vi "ZoneBlue to ZoneRed.vi"   [LabVIEW 2019]
uses:
  Global Var.vi
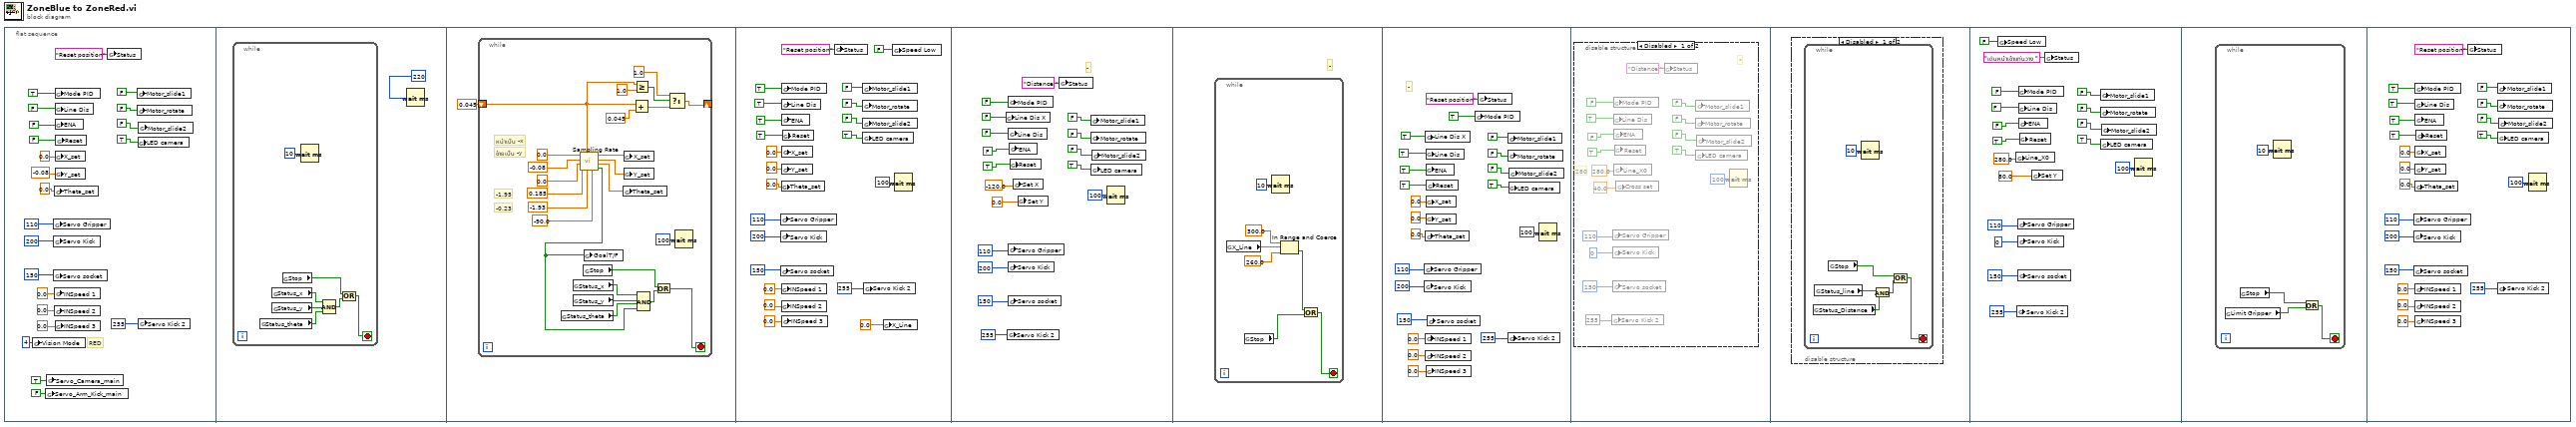
[diagram p0: block diagram]
diagram:
  n1 = flat-sequence {
    frame #0 {
      # "RED"
      n2 = global write "Global Var.vi" "Vision Mode"(i16 4 ("Vision Mode")) -> ()
      n3 = global write "Global Var.vi" "Servo_Arm_Kick_main"(FALSE ("Mode PID")) -> ()
      n4 = global write "Global Var.vi" "Servo_Camera_main"(TRUE ("Mode PID")) -> ()
      n5 = global write "Global Var.vi" "Servo Gripper"(u8 110 ("Servo Camera")) -> ()
      n6 = global write "Global Var.vi" "Servo Kick"(u8 200 ("Servo Camera")) -> ()
      n7 = global write "Global Var.vi" "Servo socket"(u8 150 ("Servo Camera")) -> ()
      n8 = global write "Global Var.vi" "Theta_set"(0.0 ("Theta_set")) -> ()
      n9 = global write "Global Var.vi" "INSpeed 1"(0.0 ("X_set")) -> ()
      n10 = global write "Global Var.vi" "INSpeed 2"(0.0 ("Y_set")) -> ()
      n11 = global write "Global Var.vi" "Mode PID"(TRUE ("Mode PID")) -> ()
      n12 = global write "Global Var.vi" "Line Dis"(FALSE ("Mode PID")) -> ()
      n13 = global write "Global Var.vi" "ENA"(FALSE ("ENA")) -> ()
      n14 = global write "Global Var.vi" "X_set"(0.0 ("X_set")) -> ()
      n15 = global write "Global Var.vi" "Y_set"(-0.08 ("Y_set")) -> ()
      n16 = global write "Global Var.vi" "INSpeed 3"(0.0 ("Theta_set")) -> ()
      n17 = global write "Global Var.vi" "Reset"(FALSE ("ENA")) -> ()
      n18 = global write "Global Var.vi" "Status"("Reset position" ("Status")) -> ()
      n19 = global write "Global Var.vi" "Motor_slide1"(FALSE ("Mode PID")) -> ()
      n20 = global write "Global Var.vi" "Motor_rotate"(FALSE ("ENA")) -> ()
      n21 = global write "Global Var.vi" "LED camera"(TRUE ("LED camera")) -> ()
      n22 = global write "Global Var.vi" "Motor_slide2"(FALSE ("ENA")) -> ()
      n23 = global write "Global Var.vi" "Servo Kick 2"(u8 255 ("Servo Camera")) -> ()
    }
    frame #1 {
      n24 = while {
        stop <- w26 stop-if-true
        n25 = global read "Global Var.vi" "Status_theta"() -> (w28:bool)
        n26 = global read "Global Var.vi" "Status_x"() -> (w29:bool)
        n27 = global read "Global Var.vi" "Status_y"() -> (w30:bool)
        n28 = global read "Global Var.vi" "Stop"() -> (w24:bool)
        n29 = Wait (ms)(milliseconds to wait=u32 10) -> ()  [unwired: 1 out]
        n30 = Compound Arithmetic op=AND(w29, w30, w28) -> (w25:bool)
        n31 = Or(x=w24, y=w25) -> (x .or. y?=w26:bool)
      }
      n32 = Wait (ms)(milliseconds to wait=u32 220) -> ()  [unwired: 1 out]
    }
    frame #2 {
      n33 = while {
        shift-right: [w34] -> _
        shift-left: 0.045 -> [w32]
        stop <- w51 stop-if-true
        # "-0.23"
        # "-1.95"
        # "ซ้ายเป็น -y"
        # "หน้าเป็น -x"
        n34 = global read "Global Var.vi" "Status_theta"() -> (w53:bool)
        n35 = global read "Global Var.vi" "Status_x"() -> (w54:bool)
        n36 = global read "Global Var.vi" "Status_y"() -> (w55:bool)
        n37 = call "Sampling Rate.vi"("input a1"=-90.0, "input y1"=-1.93, "T(0-1)"=w32, "input x1"=0.185, "input a0"=0.0, "input y0"=-0.08, "input x0"=0.0) -> ("GoalT/F"=w39:bool, "a_output"=w46:dbl, "y_output"=w47:dbl, "x_output"=w48:dbl)  [unwired: 1 in]
        n38 = global read "Global Var.vi" "Stop"() -> (w49:bool)
        n39 = global write "Global Var.vi" "GoalT/F"(w39) -> ()
        n40 = global write "Global Var.vi" "Theta_set"(w46) -> ()
        n41 = global write "Global Var.vi" "X_set"(w48) -> ()
        n42 = global write "Global Var.vi" "Y_set"(w47) -> ()
        n43 = Add(x=w32, y=0.045) -> (x+y=w37:dbl)
        n44 = Greater Or Equal?(x=w32, y=1.0) -> (x >= y?=w36:bool)
        n45 = Compound Arithmetic op=AND(w54, w55, w53, w39) -> (w50:bool)
        n46 = Or(x=w49, y=w50) -> (x .or. y?=w51:bool)
        n47 = Select(t=1.0, s=w36, f=w37) -> (s? t:f=w34:dbl)
        n48 = Wait (ms)(milliseconds to wait=u32 100) -> ()  [unwired: 1 out]
      }
    }
    frame #3 {
      n49 = global write "Global Var.vi" "Servo Gripper"(u8 110 ("Servo Camera")) -> ()
      n50 = global write "Global Var.vi" "Servo Kick"(u8 200 ("Servo Camera")) -> ()
      n51 = global write "Global Var.vi" "Servo socket"(u8 150 ("Servo Camera")) -> ()
      n52 = global write "Global Var.vi" "Theta_set"(0.0 ("Theta_set")) -> ()
      n53 = global write "Global Var.vi" "INSpeed 1"(0.0 ("X_set")) -> ()
      n54 = global write "Global Var.vi" "INSpeed 2"(0.0 ("Y_set")) -> ()
      n55 = global write "Global Var.vi" "Mode PID"(TRUE ("Mode PID")) -> ()
      n56 = global write "Global Var.vi" "Line Dis"(TRUE ("Mode PID")) -> ()
      n57 = global write "Global Var.vi" "ENA"(TRUE ("ENA")) -> ()
      n58 = global write "Global Var.vi" "X_set"(0.0 ("X_set")) -> ()
      n59 = global write "Global Var.vi" "Y_set"(0.0 ("Y_set")) -> ()
      n60 = global write "Global Var.vi" "INSpeed 3"(0.0 ("Theta_set")) -> ()
      n61 = global write "Global Var.vi" "Reset"(TRUE ("ENA")) -> ()
      n62 = global write "Global Var.vi" "Status"("Reset position" ("Status")) -> ()
      n63 = global write "Global Var.vi" "Motor_slide1"(FALSE ("Mode PID")) -> ()
      n64 = global write "Global Var.vi" "Motor_rotate"(FALSE ("ENA")) -> ()
      n65 = global write "Global Var.vi" "Motor_slide2"(FALSE ("ENA")) -> ()
      n66 = global write "Global Var.vi" "LED camera"(TRUE ("LED camera")) -> ()
      n67 = global write "Global Var.vi" "Servo Kick 2"(u8 255 ("Servo Camera")) -> ()
      n68 = global write "Global Var.vi" "X_Line"(0.0 ("X_set")) -> ()
      n69 = global write "Global Var.vi" "Speed Low"(FALSE ("LED camera")) -> ()
      n70 = Wait (ms)(milliseconds to wait=u32 100) -> ()  [unwired: 1 out]
    }
    frame #4 {
      # "-"
      n71 = global write "Global Var.vi" "Line Dis X"(FALSE ("Mode PID")) -> ()
      n72 = global write "Global Var.vi" "Servo Kick 2"(u8 255 ("Servo Camera")) -> ()
      n73 = global write "Global Var.vi" "Mode PID"(FALSE ("Mode PID")) -> ()
      n74 = global write "Global Var.vi" "Servo Gripper"(u8 110 ("Servo Camera")) -> ()
      n75 = global write "Global Var.vi" "Servo Kick"(u8 200 ("Servo Camera")) -> ()
      n76 = global write "Global Var.vi" "Servo socket"(u8 150 ("Servo Camera")) -> ()
      n77 = global write "Global Var.vi" "Line Dis"(FALSE ("Mode PID")) -> ()
      n78 = global write "Global Var.vi" "ENA"(FALSE ("ENA")) -> ()
      n79 = global write "Global Var.vi" "Reset"(TRUE ("ENA")) -> ()
      n80 = global write "Global Var.vi" "Set X"(-120.0 ("Y_set")) -> ()
      n81 = global write "Global Var.vi" "Set Y"(0.0 ("Y_set")) -> ()
      n82 = global write "Global Var.vi" "Status"("Distance " ("Status")) -> ()
      n83 = global write "Global Var.vi" "Motor_slide1"(FALSE ("Mode PID")) -> ()
      n84 = global write "Global Var.vi" "Motor_rotate"(FALSE ("ENA")) -> ()
      n85 = global write "Global Var.vi" "LED camera"(TRUE ("LED camera")) -> ()
      n86 = global write "Global Var.vi" "Motor_slide2"(FALSE ("ENA")) -> ()
      n87 = Wait (ms)(milliseconds to wait=u32 100) -> ()  [unwired: 1 out]
    }
    frame #5 {
      # "-"
      n88 = while {
        stop <- w100 stop-if-true
        n89 = global read "Global Var.vi" "X_Line"() -> (w98:dbl)
        n90 = global read "Global Var.vi" "Stop"() -> (w99:bool)
        n91 = Wait (ms)(milliseconds to wait=u32 10) -> ()  [unwired: 1 out]
        n92 = In Range and Coerce(upper limit=300.0, x=w98, lower limit=260.0) -> (In Range?=w95:bool)  [unwired: 1 out]
        n93 = Or(x=w95, y=w99) -> (x .or. y?=w100:bool)
      }
    }
    frame #6 {
      # "-"
      n94 = global write "Global Var.vi" "Servo Gripper"(u8 110 ("Servo Camera")) -> ()
      n95 = global write "Global Var.vi" "Servo Kick"(u8 200 ("Servo Camera")) -> ()
      n96 = global write "Global Var.vi" "Line Dis X"(TRUE ("Mode PID")) -> ()
      n97 = global write "Global Var.vi" "Theta_set"(0.0 ("Theta_set")) -> ()
      n98 = global write "Global Var.vi" "INSpeed 1"(0.0 ("X_set")) -> ()
      n99 = global write "Global Var.vi" "INSpeed 2"(0.0 ("Y_set")) -> ()
      n100 = global write "Global Var.vi" "Line Dis"(TRUE ("Mode PID")) -> ()
      n101 = global write "Global Var.vi" "ENA"(TRUE ("ENA")) -> ()
      n102 = global write "Global Var.vi" "X_set"(0.0 ("X_set")) -> ()
      n103 = global write "Global Var.vi" "Y_set"(0.0 ("Y_set")) -> ()
      n104 = global write "Global Var.vi" "INSpeed 3"(0.0 ("Theta_set")) -> ()
      n105 = global write "Global Var.vi" "Reset"(TRUE ("ENA")) -> ()
      n106 = global write "Global Var.vi" "Servo socket"(u8 150 ("Servo Camera")) -> ()
      n107 = global write "Global Var.vi" "Mode PID"(TRUE ("Mode PID")) -> ()
      n108 = global write "Global Var.vi" "Status"("Reset position" ("Status")) -> ()
      n109 = global write "Global Var.vi" "Motor_slide1"(FALSE ("Mode PID")) -> ()
      n110 = global write "Global Var.vi" "Motor_rotate"(FALSE ("ENA")) -> ()
      n111 = global write "Global Var.vi" "Servo Kick 2"(u8 255 ("Servo Camera")) -> ()
      n112 = global write "Global Var.vi" "LED camera"(TRUE ("LED camera")) -> ()
      n113 = global write "Global Var.vi" "Motor_slide2"(FALSE ("ENA")) -> ()
      n114 = Wait (ms)(milliseconds to wait=u32 100) -> ()  [unwired: 1 out]
    }
    frame #7 {
      n115 = disable-structure shown="Disabled" {
        frame Disabled {
          # "280"
          # "*"
          n116 = global write "Global Var.vi" "Servo Kick 2"(u8 255 ("Servo Camera")) -> ()
          n117 = global write "Global Var.vi" "Servo Gripper"(u8 110 ("Servo Camera")) -> ()
          n118 = global write "Global Var.vi" "Servo Kick"(u8 0 ("Servo Camera")) -> ()
          n119 = global write "Global Var.vi" "Servo socket"(u8 150 ("Servo Camera")) -> ()
          n120 = global write "Global Var.vi" "Mode PID"(FALSE ("Mode PID")) -> ()
          n121 = global write "Global Var.vi" "Line Dis"(TRUE ("Mode PID")) -> ()
          n122 = global write "Global Var.vi" "ENA"(FALSE ("ENA")) -> ()
          n123 = global write "Global Var.vi" "Line_X0"(280.0 ("Y_set")) -> ()
          n124 = global write "Global Var.vi" "Reset"(TRUE ("ENA")) -> ()
          n125 = global write "Global Var.vi" "Cross set"(40.0 ("Y_set")) -> ()
          n126 = global write "Global Var.vi" "Status"("Distance " ("Status")) -> ()
          n127 = global write "Global Var.vi" "Motor_slide1"(FALSE ("Mode PID")) -> ()
          n128 = global write "Global Var.vi" "Motor_rotate"(FALSE ("ENA")) -> ()
          n129 = global write "Global Var.vi" "LED camera"(TRUE ("LED camera")) -> ()
          n130 = global write "Global Var.vi" "Motor_slide2"(FALSE ("ENA")) -> ()
          n131 = Wait (ms)(milliseconds to wait=u32 100) -> ()  [unwired: 1 out]
        }
        frame Enabled {
        }
      }
    }
    frame #8 {
      n132 = disable-structure shown="Disabled" {
        frame Disabled {
          n133 = while {
            stop <- w143 stop-if-true
            n134 = global read "Global Var.vi" "Status_Distance"() -> (w139:bool)
            n135 = global read "Global Var.vi" "Status_line"() -> (w140:bool)
            n136 = global read "Global Var.vi" "Stop"() -> (w142:bool)
            n137 = Wait (ms)(milliseconds to wait=u32 10) -> ()  [unwired: 1 out]
            n138 = And(x=w140, y=w139) -> (x .and. y?=w141:bool)
            n139 = Or(x=w142, y=w141) -> (x .or. y?=w143:bool)
          }
        }
        frame Enabled {
        }
      }
    }
    frame #9 {
      n140 = global write "Global Var.vi" "Speed Low"(FALSE ("LED camera")) -> ()
      n141 = global write "Global Var.vi" "Line_X0"(280.0 ("Y_set")) -> ()
      n142 = global write "Global Var.vi" "Servo Kick 2"(u8 255 ("Servo Camera")) -> ()
      n143 = global write "Global Var.vi" "Servo Gripper"(u8 110 ("Servo Camera")) -> ()
      n144 = global write "Global Var.vi" "Servo Kick"(u8 0 ("Servo Camera")) -> ()
      n145 = global write "Global Var.vi" "Servo socket"(u8 150 ("Servo Camera")) -> ()
      n146 = global write "Global Var.vi" "Mode PID"(FALSE ("Mode PID")) -> ()
      n147 = global write "Global Var.vi" "Line Dis"(FALSE ("Mode PID")) -> ()
      n148 = global write "Global Var.vi" "ENA"(FALSE ("ENA")) -> ()
      n149 = global write "Global Var.vi" "Reset"(TRUE ("ENA")) -> ()
      n150 = global write "Global Var.vi" "Set Y"(80.0 ("Y_set")) -> ()
      n151 = global write "Global Var.vi" "Status"("เดินหน้าเข้าแท่นวาง " ("Status")) -> ()
      n152 = global write "Global Var.vi" "Motor_slide1"(FALSE ("Mode PID")) -> ()
      n153 = global write "Global Var.vi" "Motor_rotate"(FALSE ("ENA")) -> ()
      n154 = global write "Global Var.vi" "LED camera"(TRUE ("LED camera")) -> ()
      n155 = global write "Global Var.vi" "Motor_slide2"(FALSE ("ENA")) -> ()
      n156 = Wait (ms)(milliseconds to wait=u32 100) -> ()  [unwired: 1 out]
    }
    frame #10 {
      n157 = while {
        stop <- w164 stop-if-true
        n158 = global read "Global Var.vi" "Limit Gripper"() -> (w162:bool)
        n159 = global read "Global Var.vi" "Stop"() -> (w163:bool)
        n160 = Wait (ms)(milliseconds to wait=u32 10) -> ()  [unwired: 1 out]
        n161 = Or(x=w163, y=w162) -> (x .or. y?=w164:bool)
      }
    }
    frame #11 {
      n162 = global write "Global Var.vi" "Servo Gripper"(u8 110 ("Servo Camera")) -> ()
      n163 = global write "Global Var.vi" "Servo Kick"(u8 200 ("Servo Camera")) -> ()
      n164 = global write "Global Var.vi" "Servo socket"(u8 150 ("Servo Camera")) -> ()
      n165 = global write "Global Var.vi" "Theta_set"(0.0 ("Theta_set")) -> ()
      n166 = global write "Global Var.vi" "INSpeed 1"(0.0 ("X_set")) -> ()
      n167 = global write "Global Var.vi" "INSpeed 2"(0.0 ("Y_set")) -> ()
      n168 = global write "Global Var.vi" "Mode PID"(TRUE ("Mode PID")) -> ()
      n169 = global write "Global Var.vi" "Line Dis"(TRUE ("Mode PID")) -> ()
      n170 = global write "Global Var.vi" "ENA"(TRUE ("ENA")) -> ()
      n171 = global write "Global Var.vi" "X_set"(0.0 ("X_set")) -> ()
      n172 = global write "Global Var.vi" "Y_set"(0.0 ("Y_set")) -> ()
      n173 = global write "Global Var.vi" "INSpeed 3"(0.0 ("Theta_set")) -> ()
      n174 = global write "Global Var.vi" "Reset"(TRUE ("ENA")) -> ()
      n175 = global write "Global Var.vi" "Status"("Reset position" ("Status")) -> ()
      n176 = global write "Global Var.vi" "Motor_slide1"(FALSE ("Mode PID")) -> ()
      n177 = global write "Global Var.vi" "Motor_rotate"(FALSE ("ENA")) -> ()
      n178 = global write "Global Var.vi" "Servo Kick 2"(u8 255 ("Servo Camera")) -> ()
      n179 = global write "Global Var.vi" "LED camera"(TRUE ("LED camera")) -> ()
      n180 = global write "Global Var.vi" "Motor_slide2"(FALSE ("ENA")) -> ()
      n181 = Wait (ms)(milliseconds to wait=u32 100) -> ()  [unwired: 1 out]
    }
  }
